vi "InitOlfactometerValves.vi"   [LabVIEW 2016]
uses:
  <vilib>/DAQmx/write.llb/DAQmx Write.vi
  <vilib>/DAQmx/write.llb/DAQmx Write (Digital 1D Bool NChan 1Samp 1Line).vi
  <vilib>/DAQmx/create/channels.llb/DAQmx Create Channel (DO-Digital Output).vi
  <vilib>/DAQmx/miscellaneous.llb/DAQmx Fill In Error Info.vi
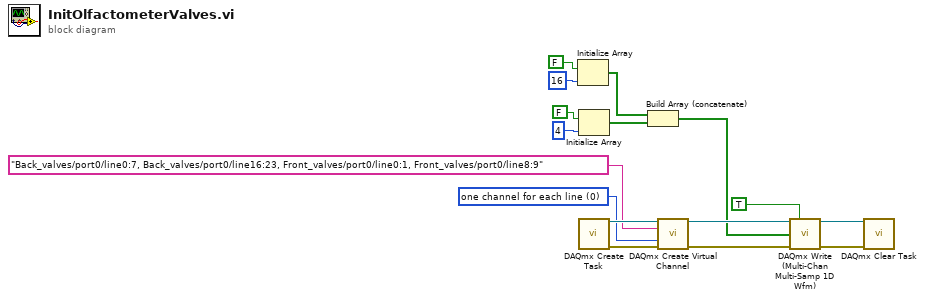
[diagram p0: block diagram]
diagram:
  w8 = 0 items=["one channel for each line", "one channel for all lines"] ("line grouping")
  n1 = Initialize Array(FALSE ("Boolean"), 16 ("dimension size")) -> (w3:bool[])
  n2 = Initialize Array(FALSE ("Boolean"), 4 ("dimension size")) -> (w2:bool[])
  n3 = call <vilib>:"DAQmx Create Task.vi"() -> ("task out"=w16:refnum<k21>, "error out"=w15:errorcluster)  [unwired: 14 in]
  n4 = Build Array (concatenate)(w3, w2) -> (w1:bool[])
  n5 = call-poly <vilib>:"DAQmx Create Virtual Channel.vi"("task in"=w16, "lines"=tag "Back_valves/port0/line0:7, Back_valves/port0/line16:23, Front_valves/port0/line0:1, Front_valves/port0/line8:9", "line grouping"=w8, "error in"=w15) -> ("task out"=w13:refnum<k21>, "error out"=w12:errorcluster)  [unwired: 10 in]
  n6 = call-poly "DAQmx Write (Multi-Chan Multi-Samp 1D Wfm).vi"("task/channels in"=w13, "auto start"=TRUE, "data"=w1, "error in"=w12) -> ("task out"=w11:refnum<k21>, "error out"=w9:errorcluster)  [unwired: 9 in, 1 out]
  n7 = call <vilib>:"DAQmx Clear Task.vi"("task in"=w11, "error in"=w9) -> ()  [unwired: 13 in, 1 out]
